vi "23384_Davis_Poku_Amankwa_Amankwa.DavisPoku.MNE1201.5.DIY_348259_723558322.vi"(10 "Path":path) -> (2 "XY CLUSTER":cluster{"x":dbl[], "y":dbl[]})   [LabVIEW 2018]
uses:
  <vilib>/Utility/file.llb/Read Delimited Spreadsheet (DBL).vi
panel:
  out "XY Graph":cluster{"all rows":dbl[], "all rows":dbl[]}(graph)
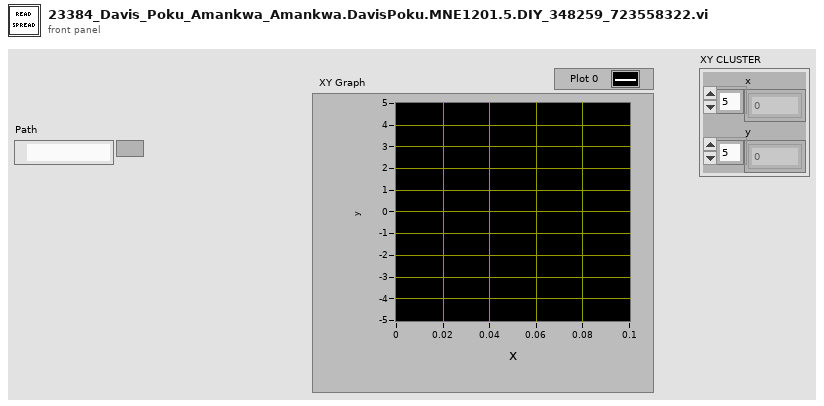
[diagram p1: front panel]
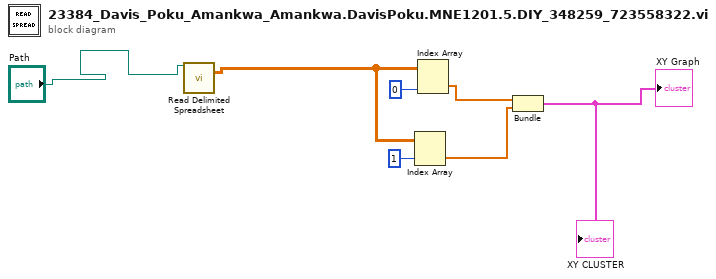
[diagram p0: block diagram]
diagram:
  n1 = call-poly <vilib>:"Read Delimited Spreadsheet.vi"("file path (dialog if empty)"="Path") -> ("all rows"=w4:dbl[][])  [unwired: 9 in, 5 out]
  n2 = Index Array(array=w4, index (col)=1) -> (element=w6:dbl[])  [unwired: 1 in]
  n3 = Index Array(array=w4, index (col)=0) -> (element=w7:dbl[])  [unwired: 1 in]
  n4 = Bundle("all rows"=w7, "all rows"=w6) -> (→"XY Graph" →"XY CLUSTER":cluster{"all rows":dbl[], "all rows":dbl[]})  [unwired: 1 in]
